vi "Rectangel Add.vi"(1 "bounds1":T1 {"height" format="%.2f"; "width" format="%.2f"; "y" format="%.2f"; "x" format="%.2f"}, 2 "bounds2":T1 {"height" format="%.2f"; "width" format="%.2f"; "y" format="%.2f"; "x" format="%.2f"}, 3 "bounds3":T1 {"height" format="%.2f"; "width" format="%.2f"; "y" format="%.2f"; "x" format="%.2f"}, 5 "error in (no error)":errorcluster, 7 "useAbsoluteCordinates(False)":bool) -> (15 "boundsAdded":T1 {"height" format="%.2f"; "width" format="%.2f"; "y" format="%.2f"; "x" format="%.2f"}, 19 "error out":errorcluster)   [LabVIEW 2012]
doc: "contains"
uses:
  <resource>/Framework/Providers/Open_GDS/UML/General/Rectangle/Rectangle Rectangle2D.ctl
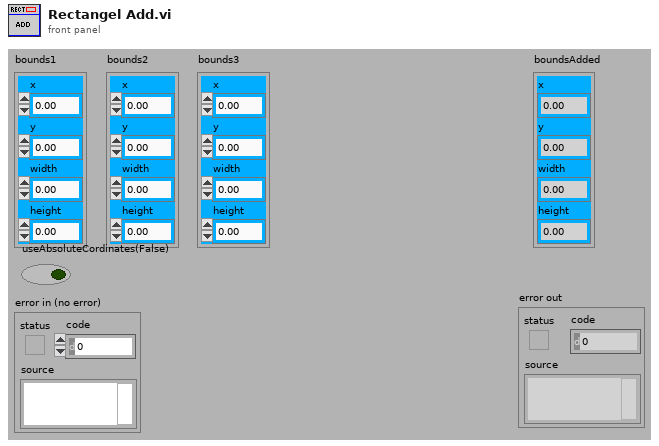
[diagram p1: front panel]
types:
  T1 = typedef "Rectangle Rectangle2D.ctl" = cluster{"x":dbl, "y":dbl, "width":dbl, "height":dbl}
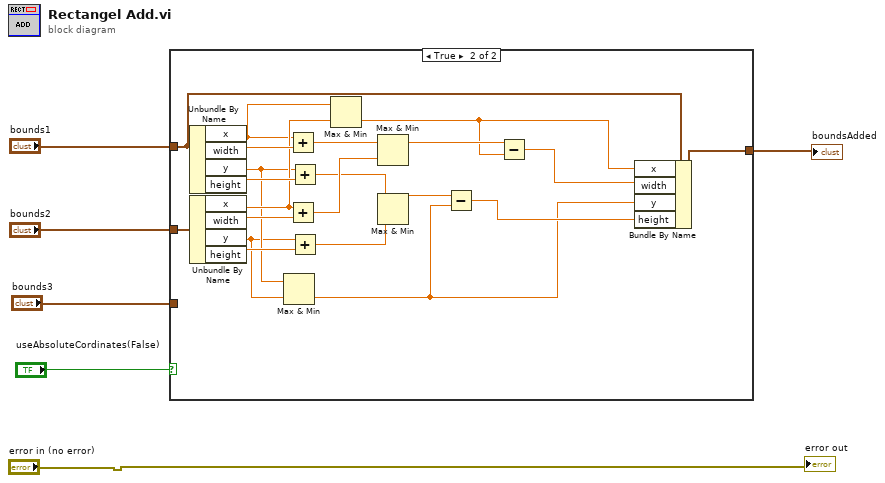
[diagram p0: block diagram]
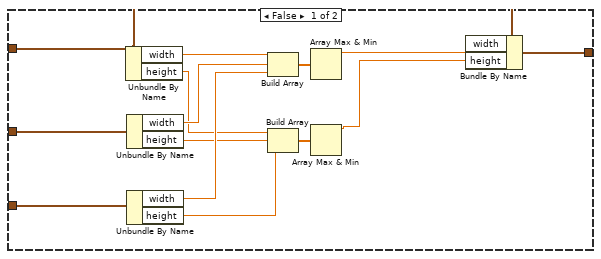
[diagram p2: hidden frame]
diagram:
  n1 = case shown="True" "useAbsoluteCordinates(False)" {
    tunnel: "bounds1" -> [w20 w32]
    tunnel: [w19 w31] -> w4
    tunnel: "bounds2" -> [w17 w36]
    tunnel: "bounds3" -> [w16 _]
    frame False {
      n2 = Unbundle By Name(w20) -> ("width"=w18:dbl, "height"=w12:dbl)
      n3 = Unbundle By Name(w17) -> ("width"=w15:dbl, "height"=w13:dbl)
      n4 = Unbundle By Name(w16) -> ("width"=w14:dbl, "height"=w11:dbl)
      n5 = Build Array(w18, w15, w14) -> (w10:dbl[])
      n6 = Build Array(w12, w13, w11) -> (w9:dbl[])
      n7 = Array Max & Min(array=w10) -> (max value=w8:dbl)  [unwired: 3 out]
      n8 = Array Max & Min(array=w9) -> (max value=w7:dbl)  [unwired: 3 out]
      n9 = Bundle By Name(cluster=w20, "width"=w8, "height"=w7) -> (w19:T1)
    }
    frame True {
      n10 = Unbundle By Name(w32) -> ("x"=w25:dbl, "width"=w41:dbl, "y"=w24:dbl, "height"=w40:dbl)
      n11 = Unbundle By Name(w36) -> ("x"=w26:dbl, "width"=w37:dbl, "y"=w23:dbl, "height"=w38:dbl)
      n12 = Max & Min(x=w24, y=w23) -> (min(x,y)=w21:dbl)  [unwired: 1 out]
      n13 = Add(x=w25, y=w41) -> (x+y=w39:dbl)
      n14 = Add(x=w26, y=w37) -> (x+y=w35:dbl)
      n15 = Add(x=w24, y=w40) -> (x+y=w34:dbl)
      n16 = Add(x=w23, y=w38) -> (x+y=w33:dbl)
      n17 = Max & Min(x=w25, y=w26) -> (min(x,y)=w22:dbl)  [unwired: 1 out]
      n18 = Max & Min(x=w39, y=w35) -> (max(x,y)=w27:dbl)  [unwired: 1 out]
      n19 = Max & Min(x=w34, y=w33) -> (max(x,y)=w29:dbl)  [unwired: 1 out]
      n20 = Subtract(x=w29, y=w21) -> (x-y=w28:dbl)
      n21 = Subtract(x=w27, y=w22) -> (x-y=w30:dbl)
      n22 = Bundle By Name(cluster=w32, "x"=w22, "width"=w30, "y"=w21, "height"=w28) -> (w31:T1)
    }
  }
  "boundsAdded" <- w4
  "error out" <- "error in (no error)"
